vi "moving avg.vi"(9 "array":dbl[](array[numeric]), 11 "no. moving avg.":i32=5) -> (2 "output array":dbl[](array[numeric]), 3 "avg.":dbl)   [LabVIEW 2018]
uses:
  <vilib>/Utility/error.llb/Error Cluster From Error Code.vi
  <vilib>/myRIO/Common/Instrument Driver Framework/myRIO v1.0/AI/vis/myRIO v1.0 Read AI.vi
  <vilib>/myRIO/Instrument Drivers/Onboard IO/AI/AI.lvlib
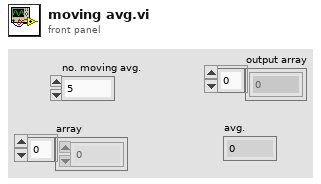
[diagram p1: front panel]
types:
  T1 = typedef "AI.lvlib/AI Reference.ctl" = cluster{"myRIO Reference":T2, "AI Channels List":T6, "AI Scaling Constants List":T8}
  T2 = typedef "myRIO Generic Hardware Reference.ctl" = cluster{"myRIO Model":T3, "myRIO Hardware Reference":T4}
  T3 = typedef "Hardware Version Enum.ctl" = enum16{"Unknown", "myRIO-1900", "myRIO-1950", "roboRIO", "NI ELVIS RIO CM", "ELVIS III"}
  T4 = typedef "myRIO v1.0 Reference.ctl" = cluster{"Generic FPGA Reference":T5, "Allow multiple opens":bool}
  T5 = typedef "Generic FPGA Reference.ctl" = refnum<k20>
  T6 = typedef "AI Channels List.ctl" = T7[]
  T7 = typedef "AI Channels Enum.ctl" = enum16{"Not Connected", "AudioIn/Left", "AudioIn/Right", "C/AI0", "C/AI1", "A/AI0", "A/AI1", "A/AI2", "A/AI3", "A/AI4", "A/AI5", "A/AI6", "A/AI7", "B/AI0", "B/AI1", "B/AI2", "B/AI3", "B/AI4", "B/AI5", "B/AI6", "B/AI7", "AI/AI0", "AI/AI1", "AI/AI2", "AI/AI3", "A/AI0 (DIFF)", "A/AI1 (DIFF)", "A/AI2 (DIFF)", "A/AI3 (DIFF)", "B/AI0 (DIFF)", "B/AI1 (DIFF)", "B/AI2 (DIFF)", "B/AI3 (DIFF)"}
  T8 = typedef "Analog Scaling Constants List.ctl" = T9[]
  T9 = typedef "Analog Scaling Constants.ctl" = cluster{"LSB Weight (Volts)":dbl, "Offset (Volts)":dbl, "Signed?":bool}
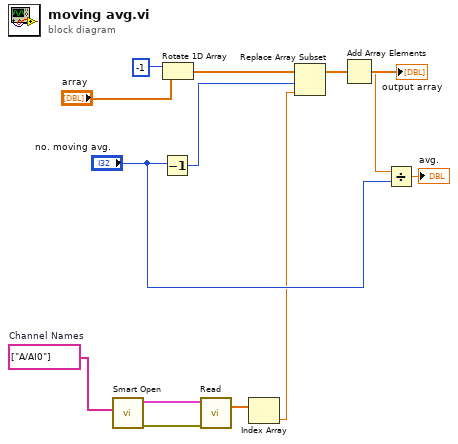
[diagram p0: block diagram]
diagram:
  w3 = tag[] ["A/AI0"]  # Channel Names
  n1 = call <vilib>:"Smart Open.vi"("Channel Names"=w3) -> ("error out"=w5:errorcluster, "AI Ref Out"=w4:T1)  [unwired: 9 in]
  n2 = Decrement(x="no. moving avg.") -> (x-1=w11:i32)
  n3 = Rotate 1D Array(1:"array", 2:-1 ("n")) -> (0:w12:dbl[])
  n4 = call <vilib>:"Read.vi"("error in (no error)"=w5, "AI Ref In"=w4) -> ("Values"=w2:dbl[])  [unwired: 7 in, 2 out]
  n5 = Index Array(array=w2) -> (element=w1:dbl)  [unwired: 1 in]
  n6 = Replace Array Subset(array=w12, new element=w1, index=w11) -> (w9:dbl[])
  "output array" <- w9
  n7 = Add Array Elements(numeric array=w9) -> (sum=w8:dbl)
  n8 = Divide(x=w8, y="no. moving avg.") -> (x/y=→"avg.":dbl)
